vi "DecodeControlRecord.vi"(11 "control record":T3={"payload data (binary string)"="\u0000\u0000\u0000\u0000\u0000\u0000\u0000\u0003", "entry ID"=1, "payload size"=0, "timestamp microSec"=0}) -> (2 "Control Record Payload Data":T2, 3 "ControlRecordType":T1)   [LabVIEW 2023]
uses:
  impl_ControlRecordType_ENUM.ctl
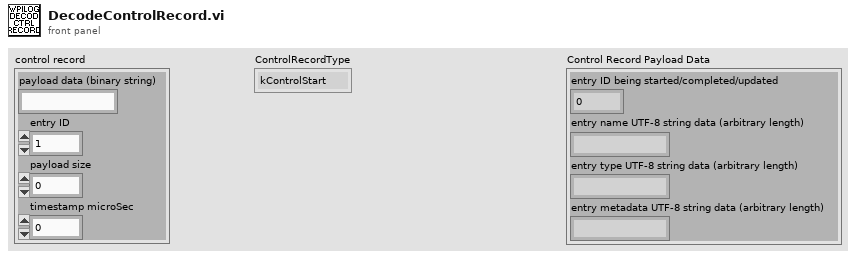
[diagram p1: front panel]
types:
  T1 = typedef "impl_ControlRecordType_ENUM.ctl" = enum16{"kControlStart", "kControlFinish", "kControlSetMetadata"}
  T2 = cluster{"entry ID being started/completed/updated":i32, "entry name UTF-8 string data (arbitrary length)":string, "entry type UTF-8 string data (arbitrary length)":string, "entry metadata UTF-8 string data (arbitrary length)":string}
  T3 = cluster{"payload data (binary string)":string, "entry ID":i32, "payload size":i32, "timestamp microSec":i32}
  T4 = enum16{"big-endian, network order", "native, host order", "little-endian"}
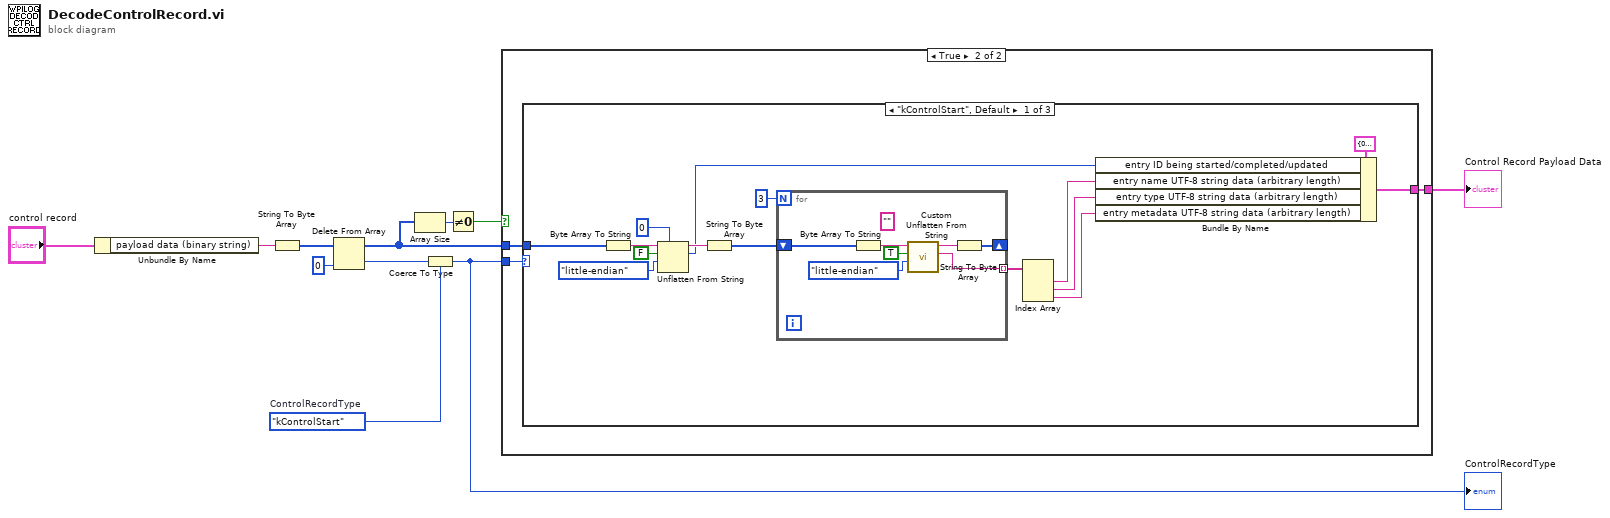
[diagram p0: block diagram]
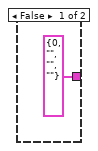
[diagram p2: hidden frame]
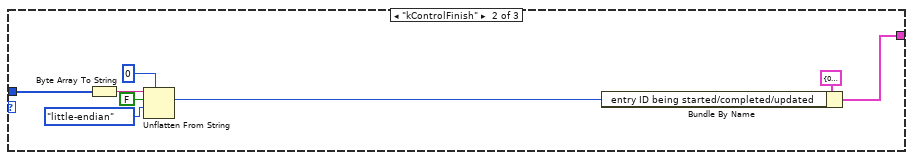
[diagram p3: hidden frame]
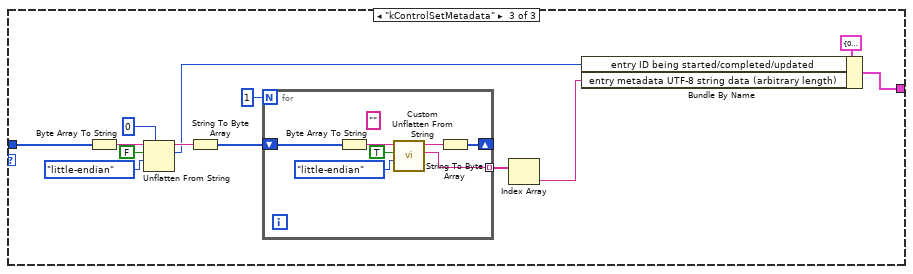
[diagram p4: hidden frame]
diagram:
  w1 = impl_ControlRecordType_ENUM."kControlStart"  # ControlRecordType
  n1 = Unbundle By Name("control record") -> ("payload data (binary string)"=w5:string)
  n2 = String To Byte Array(string=w5) -> (unsigned byte array=w9:u8[])
  n3 = Delete From Array(array=w9, index=0) -> (deleted portion=w8:u8, array with subset deleted=w4:u8[])  [unwired: 1 in]
  n4 = Array Size(array=w4) -> (size(s)=w3:i32)
  n5 = Coerce To Type(0:w8, 1:w1) -> (2:w7:T1)
  "ControlRecordType" <- w7
  n6 = Not Equal To 0?(x=w3) -> (x != 0?=w2:bool)
  n7 = case shown="True" w2 {
    tunnel: w7 -> [_ w15]
    tunnel: w4 -> [_ w14]
    tunnel: [T2 {"entry ID being started/completed/updated"=0, "entry name UTF-8 string data (arbitrary length)"="", "entry type UTF-8 string data (arbitrary length)"="", "entry metadata UTF-8 string data (arbitrary length)"=""} ("Control Record Payload Data") w13] -> w6
    frame False {
    }
    frame True {
      n8 = case shown="\"kControlStart\", Default" w15 {
        tunnel: w14 -> [w26 w42 w54]
        tunnel: [w16 w38 w47] -> w13
        frame "kControlStart", Default {
          n9 = Byte Array To String(unsigned byte array=w26) -> (string=w30:string)
          n10 = Unflatten From String(type=0, binary string=w30, data includes array or string size? (T)=FALSE, byte order (0:big-endian, network order)=T4."little-endian") -> (rest of the binary string=w27:string, value=w17:i32)  [unwired: 1 in, 1 out]
          n11 = String To Byte Array(string=w27) -> (unsigned byte array=w24:u8[])
          n12 = for {
            N: 3 -> [_]
            shift-right: [w36] -> _
            shift-left: w24 -> [w37]
            tunnel: [w33] -> w21 mode=indexing
            (unwired) ""
            n13 = Byte Array To String(unsigned byte array=w37) -> (string=w35:string)
            n14 = call "Custom Unflatten From String.vi"("byte order (0:big-endian, network order)"=T4."little-endian", "data includes array or string size? (T)"=TRUE, "binary string"=w35) -> ("value"=w33:string, "rest of the binary string"=w34:string)  [unwired: 7 in]
            n15 = String To Byte Array(string=w34) -> (unsigned byte array=w36:u8[])
          }
          n16 = Index Array(array=w21) -> (element #1=w20:string, element #2=w19:string, element #3=w18:string)  [unwired: 3 in]
          n17 = Bundle By Name(cluster=T2 {"entry ID being started/completed/updated"=0, "entry name UTF-8 string data (arbitrary length)"="", "entry type UTF-8 string data (arbitrary length)"="", "entry metadata UTF-8 string data (arbitrary length)"=""} ("Control Record Payload Data"), "entry ID being started/completed/updated"=w17, "entry name UTF-8 string data (arbitrary length)"=w20, "entry type UTF-8 string data (arbitrary length)"=w19, "entry metadata UTF-8 string data (arbitrary length)"=w18) -> (w16:T2)
        }
        frame "kControlFinish" {
          n18 = Byte Array To String(unsigned byte array=w42) -> (string=w45:string)
          n19 = Unflatten From String(type=0, binary string=w45, data includes array or string size? (T)=FALSE, byte order (0:big-endian, network order)=T4."little-endian") -> (value=w39:i32)  [unwired: 1 in, 2 out]
          n20 = Bundle By Name(cluster=T2 {"entry ID being started/completed/updated"=0, "entry name UTF-8 string data (arbitrary length)"="", "entry type UTF-8 string data (arbitrary length)"="", "entry metadata UTF-8 string data (arbitrary length)"=""} ("Control Record Payload Data"), "entry ID being started/completed/updated"=w39) -> (w38:T2)
        }
        frame "kControlSetMetadata" {
          n21 = Byte Array To String(unsigned byte array=w54) -> (string=w58:string)
          n22 = Unflatten From String(type=0, binary string=w58, data includes array or string size? (T)=FALSE, byte order (0:big-endian, network order)=T4."little-endian") -> (rest of the binary string=w55:string, value=w48:i32)  [unwired: 1 in, 1 out]
          n23 = String To Byte Array(string=w55) -> (unsigned byte array=w52:u8[])
          n24 = for {
            N: 1 -> [_]
            shift-right: [w64] -> _
            shift-left: w52 -> [w65]
            tunnel: [w61] -> w49 mode=indexing
            (unwired) ""
            n25 = Byte Array To String(unsigned byte array=w65) -> (string=w63:string)
            n26 = call "Custom Unflatten From String.vi"("byte order (0:big-endian, network order)"=T4."little-endian", "data includes array or string size? (T)"=TRUE, "binary string"=w63) -> ("value"=w61:string, "rest of the binary string"=w62:string)  [unwired: 7 in]
            n27 = String To Byte Array(string=w62) -> (unsigned byte array=w64:u8[])
          }
          n28 = Index Array(array=w49) -> (element=w46:string)  [unwired: 1 in]
          n29 = Bundle By Name(cluster=T2 {"entry ID being started/completed/updated"=0, "entry name UTF-8 string data (arbitrary length)"="", "entry type UTF-8 string data (arbitrary length)"="", "entry metadata UTF-8 string data (arbitrary length)"=""} ("Control Record Payload Data"), "entry ID being started/completed/updated"=w48, "entry metadata UTF-8 string data (arbitrary length)"=w46) -> (w47:T2)
        }
      }
    }
  }
  "Control Record Payload Data" <- w6
